vi "ReturnMovePattern.vi"(8 "error in (no error)":errorcluster, 11 "object in":refnum<class "Rook.lvclass">) -> (0 "error out":errorcluster, 3 "object out":refnum<class "Rook.lvclass">)   [LabVIEW 2020, in "Rook.lvclass"]
uses:
  Rook.lvclass
  C:/_repos/_personal/Chess/Chess_LV/source/Pieces/Piece.lvclass
  832e6eef-57f0-4f6a-956a-6b3084d6d4fb.vi
  Piece.lvclass
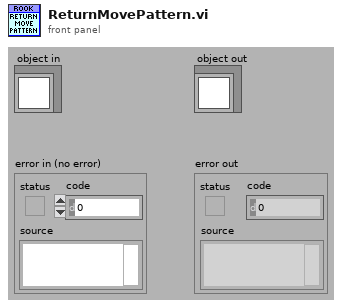
[diagram p1: front panel]
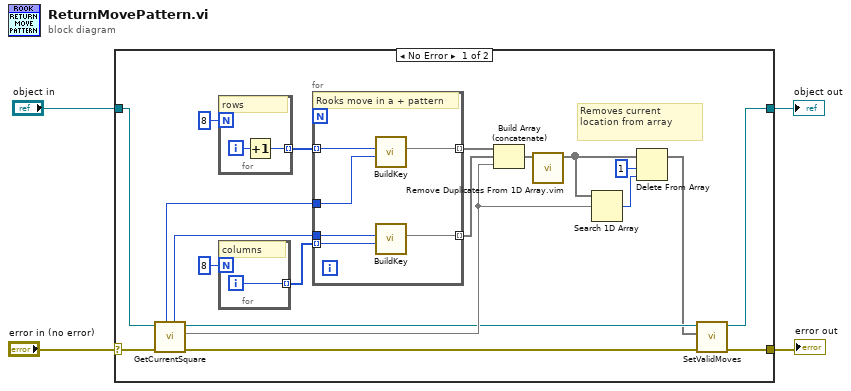
[diagram p0: block diagram]
diagram:
  n1 = case shown="No Error" "error in (no error)" {
    selector: "error in (no error)" -> [w24 w35]
    tunnel: [w10 w35] -> w3
    tunnel: [w8 w34] -> w1
    tunnel: "object in" -> [w22 w34]
    frame No Error {
      # "Removes current location from array"
      n2 = call "GetCurrentSquare.vi"("error in (no error)"=w24, "object in"=w22) -> ("error out"=w23:errorcluster, "currentSquare"=w13:map{string, i32}, "object out"=w9:refnum<class "Rook.lvclass">, "Row"=w16:i32, "Column (Numeric)"=w15:u8)  [unwired: 4 in, 1 out]
      n3 = for {
        N: 8 -> [_]
        tunnel: [w26] -> w19 mode=indexing
        i -> [w27]
        # "rows"
        n4 = Increment(x=w27) -> (x+1=w26:i32)
      }
      n5 = for {
        N: 8 -> [_]
        tunnel: [w25] -> w18 mode=indexing
        i -> [w25]
        # "columns"
      }
      n6 = for {
        tunnel: w19 -> [w33] mode=indexing
        tunnel: w18 -> [w31] mode=indexing
        tunnel: [w32] -> w17 mode=indexing
        tunnel: w16 -> [w30]
        tunnel: w15 -> [w29]
        tunnel: [w28] -> w14 mode=indexing
        # "Rooks move in a + pattern"
        n7 = call "BuildKey.vi"("Column (65=A)"=w29, "Row (>=1)"=w33) -> ("Built Key"=w32:map{string, i32})  [unwired: 7 in, 2 out]
        n8 = call "BuildKey.vi"("Column (65=A)"=w31, "Row (>=1)"=w30) -> ("Built Key"=w28:map{string, i32})  [unwired: 7 in, 2 out]
      }
      n9 = Build Array (concatenate)(w17, w14, w13) -> (w6:map{string, i32}[])
      n10 = call "Remove Duplicates From 1D Array.vim"("array"=w6) -> ("array with duplicates removed"=w5:map{string, i32}[])  [unwired: 10 in]
      n11 = Search 1D Array(1D array=w5, element=w13) -> (index of element=w11:i32)  [unwired: 1 in]
      n12 = Delete From Array(array=w5, length=1, index=w11) -> (array with subset deleted=w7:map{string, i32}[])  [unwired: 1 out]
      n13 = call "SetValidMoves.vi"("error in (no error)"=w23, "validMoves"=w7, "object in"=w9) -> ("error out"=w10:errorcluster, "object out"=w8:refnum<class "Rook.lvclass">)  [unwired: 7 in]
    }
    frame Error {
    }
  }
  "error out" <- w3
  "object out" <- w1
